vi "uTTA_Read_T3rFile.vi"(8 "error in":errorcluster, 11 "File Path":path) -> (0 "error out":errorcluster, 1 "RunTime":dbl, 3 "T3R-File":string)   [LabVIEW 2021]
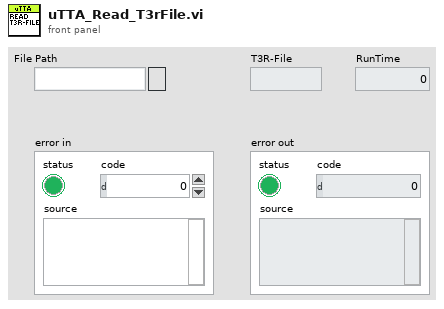
[diagram p1: front panel]
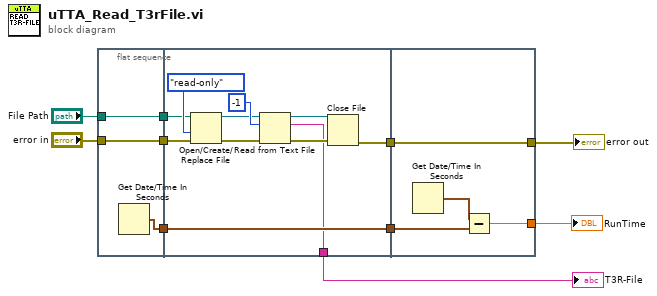
[diagram p0: block diagram]
diagram:
  n1 = flat-sequence {
    tunnel: "File Path" -> [w12]
    tunnel: "error in" -> [w13]
    tunnel: [w13] -> w7
    tunnel: [w12] -> w6
    tunnel: [w11] -> w4
    tunnel: w7 -> [w17]
    tunnel: w6 -> [w16]
    tunnel: [w24] -> w5
    tunnel: w4 -> [w15]
    tunnel: [w15] -> w3
    tunnel: [w14] -> w2
    tunnel: [w28] -> w10
    tunnel: w5 -> [w28]
    tunnel: w3 -> [w26]
    tunnel: [w25] -> w1
    frame #0 {
      n2 = Get Date/Time In Seconds() -> (seconds since 1Jan1904=w11:timestamp)
    }
    frame #1 {
      n3 = Open/Create/Replace File(file path (use dialog)=w16, error in=w17, access (0:read/write)=enum16{"read/write", "read-only", "write-only"}."read-only") -> (refnum out=w19:refnum<file>, error out=w20:errorcluster)  [unwired: 3 in, 1 out]
      n4 = Read from Text File(file (use dialog)=w19, count=-1, error in=w20) -> (refnum out=w22:refnum<file>, text=w14:string, error out=w23:errorcluster)  [unwired: 1 in, 1 out]
      n5 = Close File(refnum=w22, error in=w23) -> (error out=w24:errorcluster)  [unwired: 1 out]
    }
    frame #2 {
      n6 = Get Date/Time In Seconds() -> (seconds since 1Jan1904=w27:timestamp)
      n7 = Subtract(x=w27, y=w26) -> (x-y=w25:dbl)
    }
  }
  "error out" <- w10
  "T3R-File" <- w2
  "RunTime" <- w1
